vi "Input First Hour Settings.vi"(7 "GEA2 HyperData":bool=TRUE, 9 "COM Port":refnum<visa-resource-name>="COM3", 11 "Heating  Mode":T2=enum."Hybrid Heating") -> (4 "GEA2 Set Mode Out":T1=enum."HighDemand", 6 "Set PointOut":u8=140, 8 "GEA2 HyperData Out":bool, 10 "COM Port Out":refnum<visa-resource-name>="COM3", 15 "Heating  Mode Out":T2=enum."Hybrid Heating")   [LabVIEW 2009]
uses:
  Heating Modes.ctl
  GEA2/HEWH_Mode.ctl
panel:
  in  "Set Point":u8=140
  in  "Complete":bool
  # "1st Hour Test Setup"
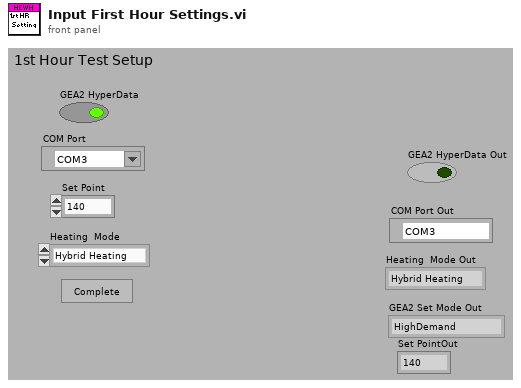
[diagram p1: front panel]
types:
  T1 = typedef "HEWH_Mode.ctl" = enum16{"Hybrid", "StdElectric", "eHeat", "HighDemand", "Unknown"}
  T2 = typedef "Heating Modes.ctl" = enum16{"Standard Electric", "Hybrid Heating", "E-Heat Mode"}
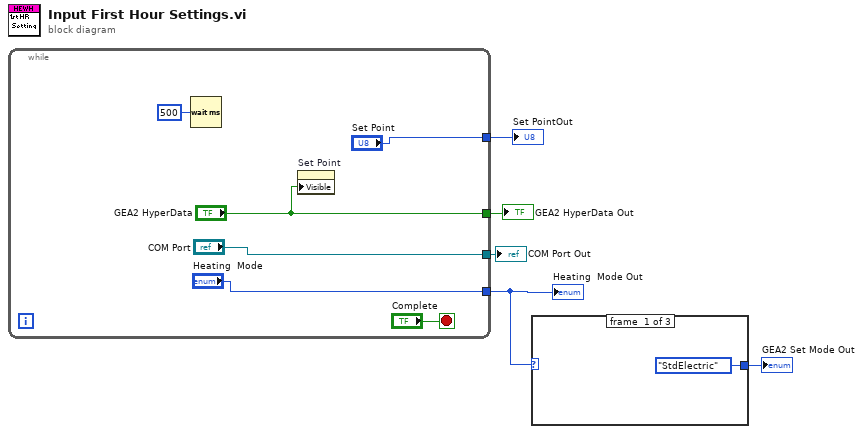
[diagram p0: block diagram]
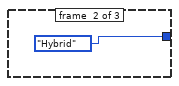
[diagram p2: hidden frame]
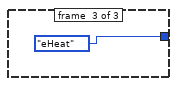
[diagram p3: hidden frame]
diagram:
  n1 = while {
    tunnel: ["GEA2 HyperData"] -> w5
    tunnel: ["COM Port"] -> w4
    tunnel: ["Heating  Mode"] -> w2
    tunnel: ["Set Point"] -> w3
    stop <- "Complete" stop-if-true
    n2 = Wait (ms)(milliseconds to wait=u32 500) -> ()  [unwired: 1 out]
    n3 = property on="Set Point" class="DigNum (strict)"("Visible"="GEA2 HyperData") -> ()  [unwired: 2 in, 2 out]
  }
  "COM Port Out" <- w4
  "GEA2 HyperData Out" <- w5
  "Heating  Mode Out" <- w2
  "Set PointOut" <- w3
  n4 = case shown="\"E-Heat Mode\"" w2 {
    tunnel: [HEWH_Mode."StdElectric" ("Mode Out") HEWH_Mode."Hybrid" ("Mode Out") HEWH_Mode."eHeat" ("Mode Out")] -> w1
    frame #0 {
    }
    frame #1 {
    }
    frame #2 {
    }
  }
  "GEA2 Set Mode Out" <- w1
